vi "PartialCluster4.vi"(3 "Cluster1":T2) -> (0 "A * B":T1)   [LabVIEW 2011]
uses:
  <vilib>/Analysis/Matrix/Datatypes/RealMatrix.ctl
  <vilib>/Analysis/Matrix/Numeric/Multiply/Multiply - RM,RM.vi
  <vilib>/Analysis/Matrix/NI_Matrix.lvlib
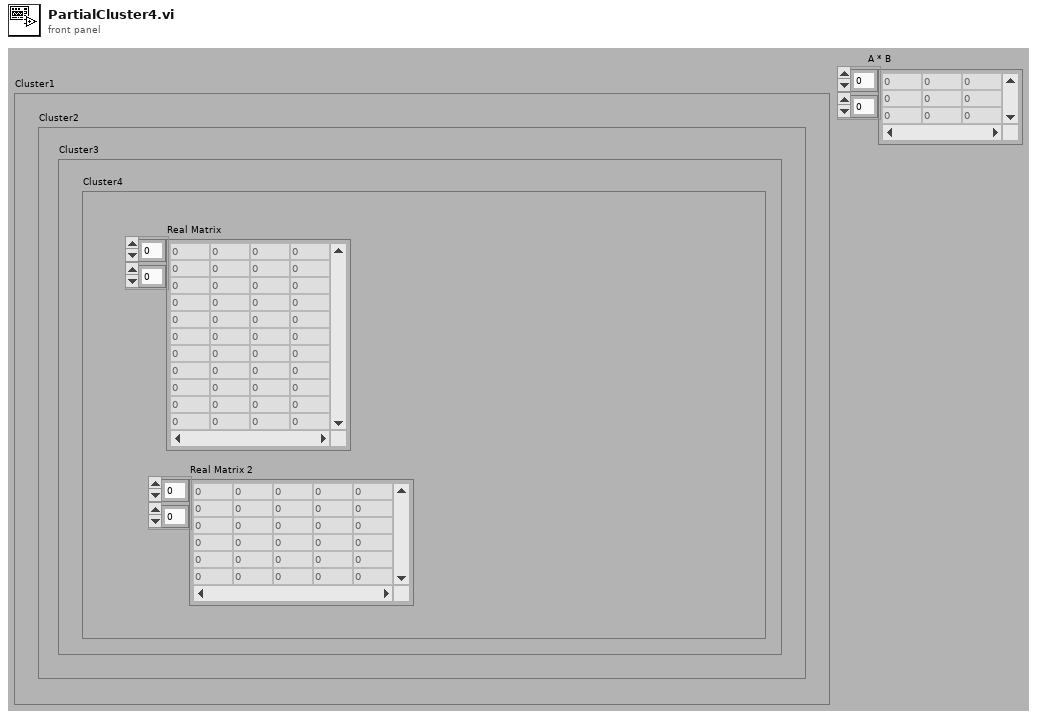
[diagram p1: front panel]
types:
  T1 = typedef "NI_Matrix.lvlib/RealMatrix.ctl" = dbl[][]
  T2 = cluster{"Cluster2":cluster{"Cluster3":cluster{"Cluster4":cluster{"Real Matrix":T1, "Real Matrix 2":T1}}}}
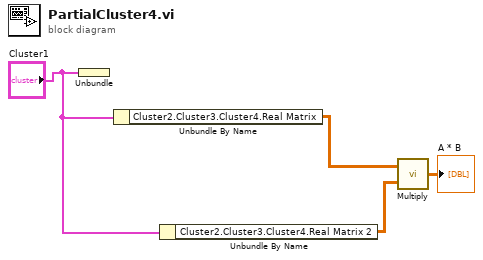
[diagram p0: block diagram]
diagram:
  n1 = Unbundle("Cluster1") -> ()  [unwired: 1 out]
  n2 = Unbundle By Name("Cluster1") -> ("Cluster2.Cluster3.Cluster4.Real Matrix"=w3:T1)
  n3 = Unbundle By Name("Cluster1") -> ("Cluster2.Cluster3.Cluster4.Real Matrix 2"=w2:T1)
  n4 = call-poly <vilib>:"Multiply.vi"("Real Matrix B"=w2, "Real Matrix A"=w3) -> ("A * B"=→"A * B":T1)
